vi "Main_05B.vi"() -> ()   [LabVIEW 2025]
uses:
  Utility/Universal Utility/TypeDefs_Utility/Cluster_Row-Column.ctl
  9e3f57c0-2ef8-4495-8287-c6a42a5fb955.vi
  Utility/Universal Utility/TypeDefs_Utility/ENUM_4 Directions U-D-L-R.ctl
  Utility/Universal Utility/TypeDefs_Utility/ENUM_8 Directions U-D-L-R.ctl
panel:
  out "Min":u64[](array[numeric])
  out "max":u64[](array[numeric])
  out "x-1":u64
  out "MATCH":bool
  in  "Select Data":enum32{"Example", "test", "Puzzle"}(tab)
  in  "EX Target":u32=14
  in  "Example":string="3-5\n10-14\n16-20\n12-18\n\n1\n5\n8\n11\n17\n32"
  in  "test":u32=40
  in  "test":string="3-5\n10-14\n16-20\n12-18\n\n1\n5\n8\n11\n17\n32"
  in  "Puzzle":string="505104443555011-505832008521290\n183705568221799-189071596736306\n25714421842394-26498060657296\n324591982604436-326326266144576\n194954655268286-199771011784310\n32539515377401-39552166142220\n326326266144577-330576407995732\n45877724695638-45877724695638\n245990755269494-248893742631986\n316826876448244-321016747706186\n23726069480801-24221552311396\n282687875186245-282687875186245\n84944235636755-86138442862850\n27463398169403-27981167005022\n388889831860114-389071080230049\n178876097666360-180498038018267\n509753176570993-510393291709325\n137682268842164-139478866740539\n504458187396917-505104443555011\n5030..."
  in  "Puzzle Target":u32
  out "Answer":u64
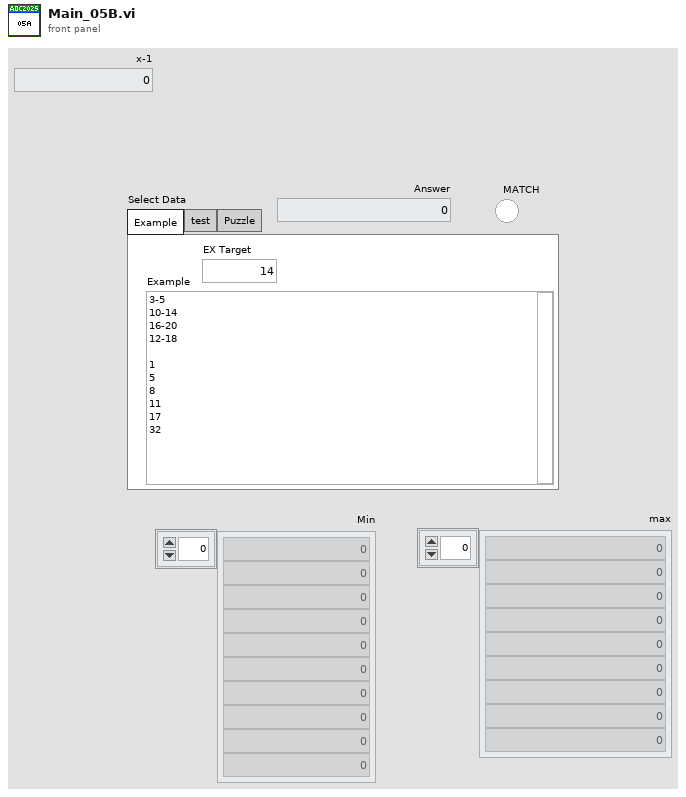
[diagram p1: front panel]
types:
  T1 = typedef "ENUM_8 Directions U-D-L-R.ctl" = enum16{"Up;-1,0", "Up-Right;-1,1", "Right;0,1", "Down-Right;1,1", "Down;1,0", "Down-Left;1,-1", "Left;0,-1", "Up-Left;-1,-1"}
  T2 = typedef "ENUM_4 Directions U-D-L-R.ctl" = enum16{"Up;-1,0", "Right;0,1", "Down;1,0", "Left;0,-1"}
  T3 = typedef "Cluster_Row-Column.ctl" = cluster{"R":i32, "C":i32}
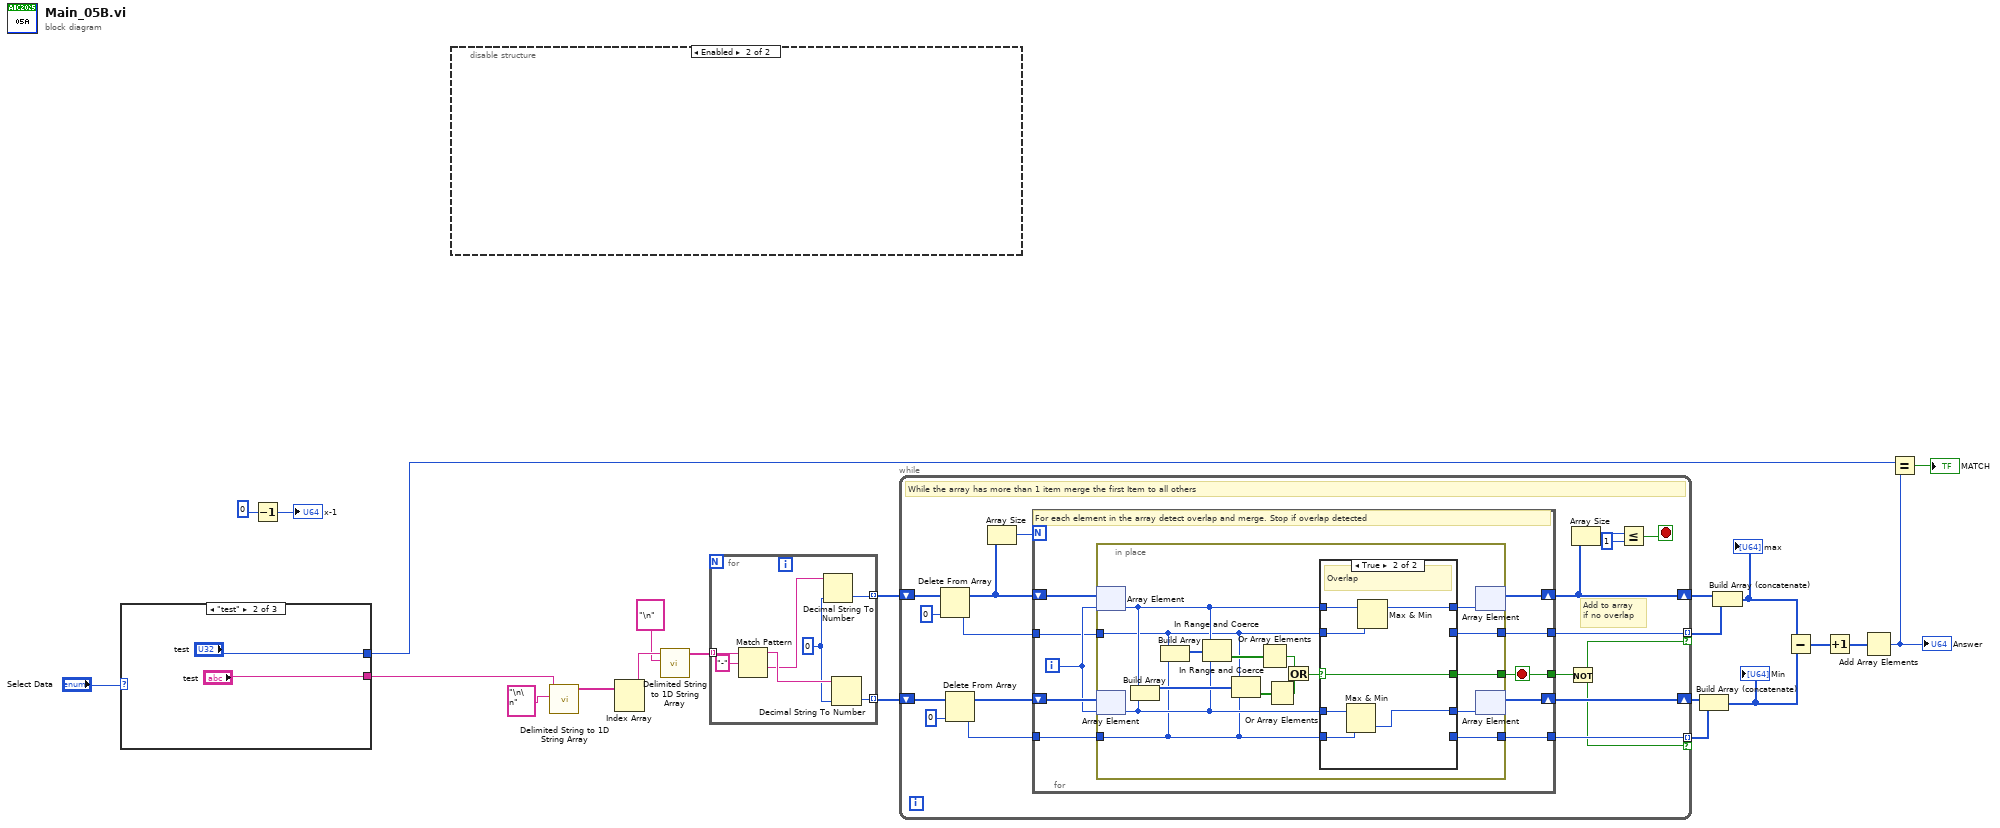
[diagram p0: block diagram]
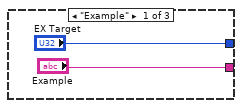
[diagram p3: hidden frame]
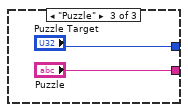
[diagram p4: hidden frame]
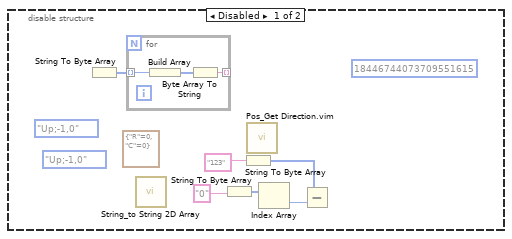
[diagram p5: hidden frame]
diagram:
  n1 = case shown="\"test\"" "Select Data" {
    tunnel: ["Example" "test" "Puzzle"] -> w21
    tunnel: ["EX Target" "test" "Puzzle Target"] -> w18
    frame "Example" {
    }
    frame "test" {
    }
    frame "Puzzle" {
    }
  }
  n2 = Decrement(x=u64 0) -> (x-1=→"x-1":u64)
  n3 = disable-structure shown="Enabled" {
    frame Disabled {
      (unwired) u64 18446744073709551615 ("x-1")
      (unwired) ENUM_8_Directions_U-D-L-R."Up;-1,0" ("Direction 8")
      (unwired) ENUM_4_Directions_U-D-L-R."Up;-1,0" ("Direction")
      (unwired) T3 {"R"=0, "C"=0} ("Position")
      n4 = String To Byte Array() -> (unsigned byte array=w29:u8[])  [unwired: 1 in]
      n5 = for {
        tunnel: w29 -> [w37] mode=indexing
        tunnel: [w35] -> _ mode=indexing
        n6 = Build Array(w37) -> (w36:u8[])
        n7 = Byte Array To String(unsigned byte array=w36) -> (string=w35:string)
      }
      n8 = call "String_to String 2D Array.vi"() -> ()  [unwired: 11 in, 1 out]
      n9 = String To Byte Array(string="0") -> (unsigned byte array=w32:u8[])
      n10 = String To Byte Array(string="123") -> (unsigned byte array=w30:u8[])
      n11 = call "Pos_Get Direction.vim"() -> ()  [unwired: 11 in, 1 out]
      n12 = Index Array(array=w32) -> (element=w31:u8)  [unwired: 1 in]
      n13 = Subtract(x=w30, y=w31) -> ()  [unwired: 1 out]
    }
    frame Enabled {
    }
  }
  n14 = call <vilib>:"Delimited String to 1D String Array.vi"("delimiter"="\n\n" ("delimiter (Tab)"), "delimited string"=w21) -> ("string array"=w15:string[])  [unwired: 9 in]
  n15 = Index Array(array=w15) -> (element #1=w14:string)  [unwired: 2 in, 1 out]
  n16 = call <vilib>:"Delimited String to 1D String Array.vi"("delimiter"="\n" ("delimiter (Tab)"), "delimited string"=w14) -> ("string array"=w12:string[])  [unwired: 9 in]
  n17 = for {
    tunnel: w12 -> [w44] mode=indexing
    tunnel: [w39] -> w9 mode=indexing
    tunnel: [w38] -> w10 mode=indexing
    w40 = u64 0 ("default (0 I32)")
    n18 = Match Pattern(string=w44, regular expression="-") -> (before substring=w42:string, after substring=w41:string)  [unwired: 1 in, 2 out]
    n19 = Decimal String To Number(string=w41, default (0L)=w40) -> (number=w39:u64)  [unwired: 1 in, 1 out]
    n20 = Decimal String To Number(string=w42, default (0L)=w40) -> (number=w38:u64)  [unwired: 1 in, 1 out]
  }
  n21 = while {
    shift-right: [w48] -> w8
    shift-left: w9 -> [w62]
    shift-right: [w53] -> w6
    shift-left: w10 -> [w61]
    tunnel: [w52] -> w7 mode=indexing if=w49
    tunnel: [w51] -> w5 mode=indexing if=w49
    stop <- w45 stop-if-true
    # "Add to array\nif no overlap"
    # "While the array has more than 1 item merge the first Item to all others"
    n22 = Delete From Array(array=w62, index=0) -> (deleted portion=w56:u64, array with subset deleted=w55:u64[])  [unwired: 1 in]
    n23 = Delete From Array(array=w61, index=0) -> (deleted portion=w57:u64, array with subset deleted=w58:u64[])  [unwired: 1 in]
    n24 = Array Size(array=w55) -> (size(s)=w54:i32)
    n25 = for {
      N: w54 -> [_]
      tunnel: w57 -> [w69]
      tunnel: w56 -> [w68]
      shift-right: [w67] -> w48
      shift-left: w55 -> [w72]
      shift-right: [w66] -> w53
      shift-left: w58 -> [w71]
      tunnel: [w65] -> w52
      tunnel: [w64] -> w51
      tunnel: [w63] -> w50
      i -> [w70]
      stop <- w63 stop-if-true
      # "For each element in the array detect overlap and merge. Stop if overlap detected"
      n26 = in-place {
        in-place-border: w69 -> [w76]
        in-place-border: w68 -> [w75]
        in-place-border: [w77] -> w63
        in-place-border: [w74] -> w65
        in-place-border: [w73] -> w64
        n27 = in-place-array #1(w72, w70) -> (w81:u64)
        n28 = in-place-array #2(w71, w70) -> (w79:u64)
        n29 = Build Array(w81, w79) -> (w87:u64[])
        n30 = Build Array(w75, w76) -> (w88:u64[])
        n31 = In Range and Coerce(upper limit=w81, x=w88, lower limit=w79) -> (In Range?=w86:bool[])  [unwired: 1 out]
        n32 = In Range and Coerce(upper limit=w75, x=w87, lower limit=w76) -> (In Range?=w85:bool[])  [unwired: 1 out]
        n33 = Or Array Elements(Boolean array=w86) -> (logical OR=w84:bool)
        n34 = Or Array Elements(Boolean array=w85) -> (logical OR=w83:bool)
        n35 = Or(x=w84, y=w83) -> (x .or. y?=w82:bool)
        n36 = case shown="True" w82 {
          selector: w82 -> [w91 w97]
          tunnel: w81 -> [w93 w100]
          tunnel: [w93 w98] -> w80
          tunnel: w79 -> [w92 w96]
          tunnel: [w92 w94] -> w78
          tunnel: [w91 w97] -> w77
          tunnel: w76 -> [w89 w95]
          tunnel: w75 -> [w90 w99]
          tunnel: [w90 _] -> w74
          tunnel: [w89 _] -> w73
          frame False {
            # "NO Overlap"
          }
          frame True {
            # "Overlap"
            n37 = Max & Min(x=w96, y=w95) -> (min(x,y)=w94:u64)  [unwired: 1 out]
            n38 = Max & Min(x=w100, y=w99) -> (max(x,y)=w98:u64)  [unwired: 1 out]
          }
        }
        n39 = in-place-array #1(w80) -> (w67:u64[])  [unwired: 1 out]
        n40 = in-place-array #2(w78) -> (w66:u64[])  [unwired: 1 out]
      }
    }
    n41 = Not(x=w50) -> (.not. x?=w49:bool)
    n42 = Array Size(array=w48) -> (size(s)=w47:i32)
    n43 = Less Or Equal?(x=w47, y=1) -> (x <= y?=w45:bool)
  }
  n44 = Build Array (concatenate)(w6, w5) -> (w2:u64[])
  "Min" <- w2
  n45 = Build Array (concatenate)(w8, w7) -> (w3:u64[])
  "max" <- w3
  n46 = Subtract(x=w3, y=w2) -> (x-y=w4:u64[])
  n47 = Increment(x=w4) -> (x+1=w1:u64[])
  n48 = Add Array Elements(numeric array=w1) -> (sum=w11:u64)
  "Answer" <- w11
  n49 = Equal?(x=w18, y=w11) -> (x = y?=→"MATCH":bool)
